vi "Wait For Stage.vi"(8 "error in (no error)":errorcluster, 10 "Target Position":dbl[](array[numeric]), 11 "Stage Readout Notifier":refnum<notifier>) -> (0 "error out":errorcluster, 2 "In Position":bool)   [LabVIEW 2015, in "XYZStage.lvlib"]
uses:
  XYZStage.lvlib
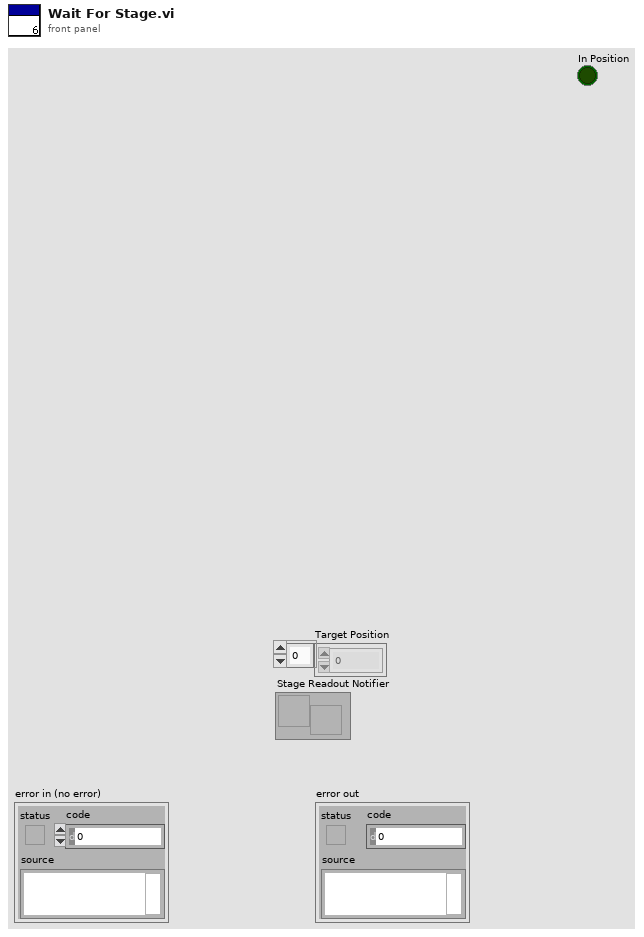
[diagram p1: front panel]
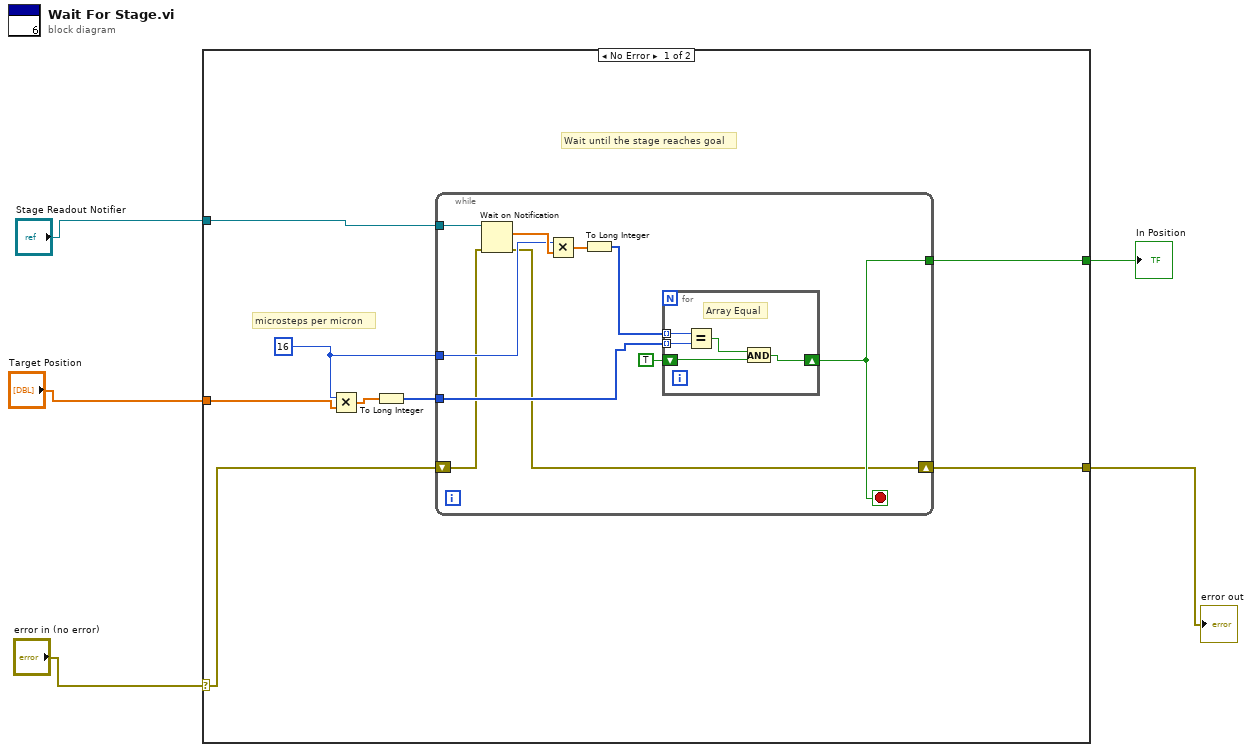
[diagram p0: block diagram]
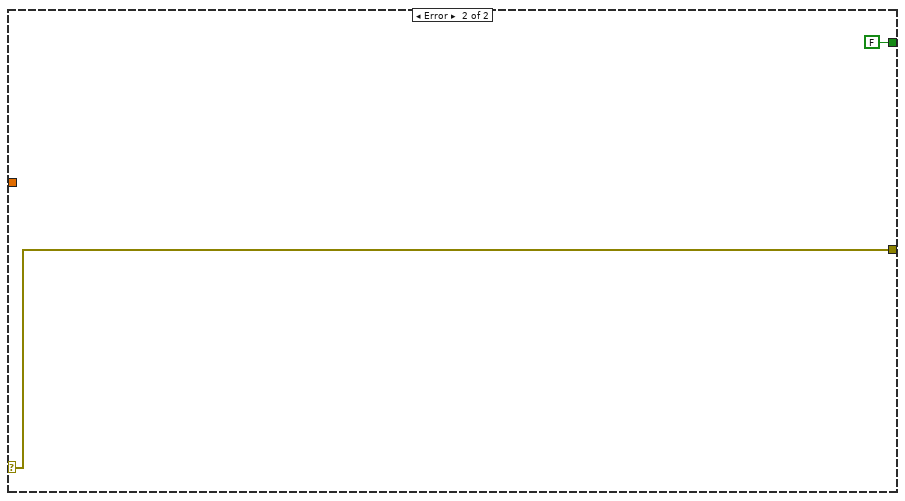
[diagram p2: hidden frame]
diagram:
  n1 = case shown="No Error" "error in (no error)" {
    selector: "error in (no error)" -> [w8 w30]
    tunnel: "Target Position" -> [w13 _]
    tunnel: "Stage Readout Notifier" -> [w12 _]
    tunnel: [w7 w30] -> w2
    tunnel: [w6 FALSE] -> w1
    frame No Error {
      w10 = 16
      # "Wait until the stage reaches goal"
      # "microsteps per micron"
      n2 = Multiply(x=w10, y=w13) -> (x*y=w11:dbl[])
      n3 = To Long Integer(number=w11) -> (32bit integer=w9:i32[])
      n4 = while {
        tunnel: w12 -> [w23]
        tunnel: w10 -> [w21]
        tunnel: w9 -> [w20]
        shift-right: [w14] -> w7
        shift-left: w8 -> [w15]
        tunnel: [w16] -> w6
        stop <- w16 stop-if-true
        n5 = Wait on Notification(notifier=w23, error in (no error)=w15) -> (notification=w22:dbl[], error out=w14:errorcluster)  [unwired: 2 in, 2 out]
        n6 = Multiply(x=w21, y=w22) -> (x*y=w19:dbl[])
        n7 = To Long Integer(number=w19) -> (32bit integer=w18:i32[])
        n8 = for {
          tunnel: w20 -> [w28] mode=indexing
          tunnel: w18 -> [w27] mode=indexing
          shift-right: [w24] -> w16
          shift-left: TRUE -> [w25]
          # "Array Equal"
          n9 = Equal?(x=w27, y=w28) -> (x = y?=w26:bool)
          n10 = And(x=w26, y=w25) -> (x .and. y?=w24:bool)
        }
      }
    }
    frame Error {
    }
  }
  "error out" <- w2
  "In Position" <- w1
